vi "ExtractSpectralInfo.vi"(8 "PeakHalfBandwidth":dbl=5.0, 9 "Min":dbl, 10 "Max":dbl, 11 "Spectrum":T1) -> (0 "Analysis":string[](array[string]), 1 "baseline":dbl format="%#_2g", 2 "peak":dbl format="%#_2g", 3 "fitCentre":dbl)   [LabVIEW 2014]
uses:
  <vilib>/Analysis/NI_AALPro.lvlib
  <vilib>/Analysis/NI_AALBase.lvlib
panel:
  in  "BaselineSmoothing":i32=200
  out "XY Graph":cluster{dbl[], "Best Gaussian Fit":dbl[]}[](graph)
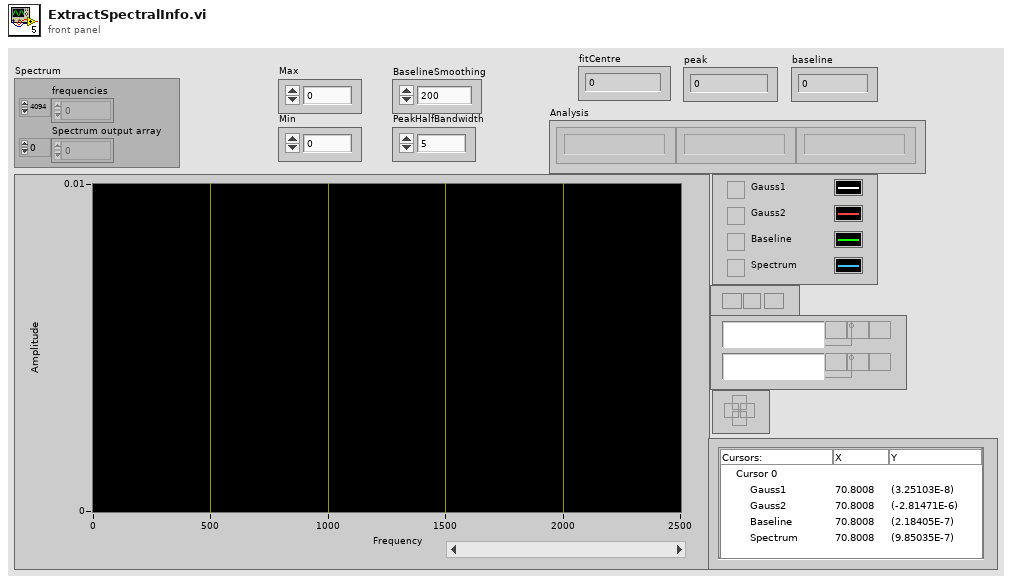
[diagram p1: front panel]
types:
  T1 = cluster{"frequencies":dbl[], "Spectrum output array":dbl[]}
  T2 = cluster{"FrequencySubset":dbl[], "Best Gaussian Fit":dbl[]}
  T3 = cluster{"frequencies":dbl[], "Spectrum output array":dbl[]}[]
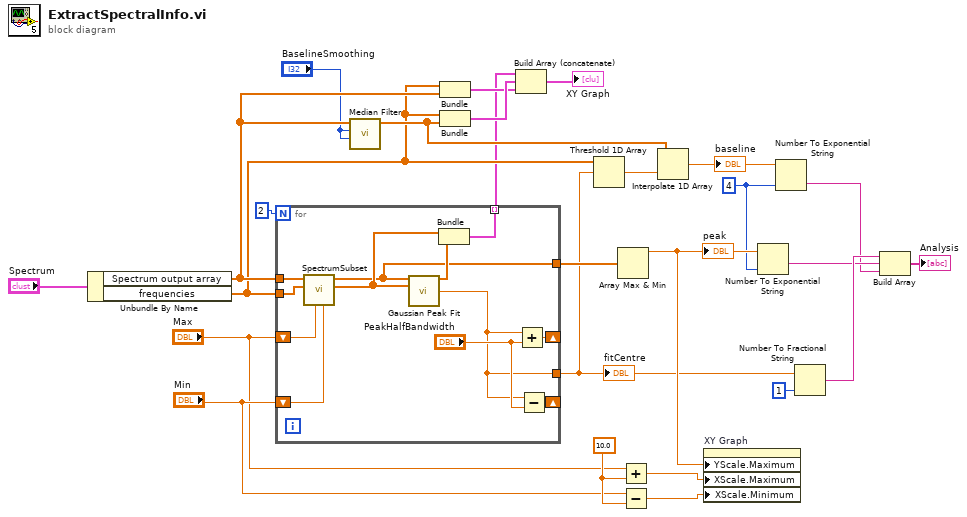
[diagram p0: block diagram]
diagram:
  w2 = i16 4 ("precision (6)")
  w13 = 10.0
  n1 = Unbundle By Name("Spectrum") -> ("Spectrum output array"=w20:dbl[], "frequencies"=w19:dbl[])
  n2 = for {
    N: 2 -> [_]
    tunnel: w20 -> [w38]
    tunnel: w19 -> [w37]
    shift-right: [w36] -> _
    shift-left: "Max" -> [w28]
    shift-right: [w35] -> _
    shift-left: "Min" -> [w27]
    tunnel: [w33] -> w7
    tunnel: [w29] -> w24
    tunnel: [w32] -> w16 mode=indexing
    n3 = call "SpectrumSubset.vi"("SearchBandMin"=w27, "SearchBandMax"=w28, "Frequencies"=w37, "Spectrum"=w38) -> ("FrequencySubset"=w31:dbl[], "SpectrumSubset"=w29:dbl[])  [unwired: 6 in]
    n4 = call <vilib>:"Gaussian Peak Fit.vi"("Y"=w29, "X"=w31) -> ("Best Gaussian Fit"=w30:dbl[], "center"=w33:dbl)  [unwired: 7 in, 5 out]
    n5 = Bundle("FrequencySubset"=w31, "Best Gaussian Fit"=w30) -> (w32:T2)  [unwired: 1 in]
    n6 = Add(x=w33, y="PeakHalfBandwidth") -> (x+y=w36:dbl)
    n7 = Subtract(x=w33, y="PeakHalfBandwidth") -> (x-y=w35:dbl)
  }
  "fitCentre" <- w7
  n8 = call <vilib>:"Median Filter.vi"("right rank"="BaselineSmoothing", "left rank"="BaselineSmoothing", "X"=w20) -> ("Filtered X"=w21:dbl[])  [unwired: 7 in, 1 out]
  n9 = Bundle("frequencies"=w19, "Spectrum output array"=w20) -> (w17:T1)  [unwired: 1 in]
  n10 = Bundle("frequencies"=w19, "Filtered X"=w21) -> (w18:cluster{"frequencies":dbl[], "Filtered X":dbl[]})  [unwired: 1 in]
  n11 = Build Array (concatenate)(w16, w18, w17) -> (→"XY Graph":T3)
  n12 = Threshold 1D Array(2:w7, 3:w19) -> (0:w22:dbl)  [unwired: 1 in]
  n13 = Array Max & Min(array=w24) -> (max value=w8:dbl)  [unwired: 3 out]
  "peak" <- w8
  n14 = Add(x="Max", y=w13) -> (x+y=w15:dbl)
  n15 = Subtract(x="Min", y=w13) -> (x-y=w14:dbl)
  n16 = Interpolate 1D Array(1:w22, 2:w21) -> (0:w9:dbl)
  "baseline" <- w9
  n17 = property on="XY Graph" class="XYGraph (strict)"("YScale.Maximum"=w8, "XScale.Maximum"=w15, "XScale.Minimum"=w14) -> ()  [unwired: 2 in, 2 out]
  n18 = Number To Exponential String(number=w8, precision (6)=w2) -> (E-format string=w5:string)  [unwired: 2 in]
  n19 = Number To Exponential String(number=w9, precision (6)=w2) -> (E-format string=w4:string)  [unwired: 2 in]
  n20 = Number To Fractional String(number=w7, precision (6)=i16 1) -> (F-format string=w6:string)  [unwired: 2 in]
  n21 = Build Array(w6, w5, w4) -> (→"Analysis":string[])
